vi "Create Interlocked Q Class.vi"(10 "Process State Data":refnum<data-value>, 11 "Process Q":refnum<class "Message Enqueuer.lvclass">) -> (3 "Interlock Q Class out":refnum<class "Interlock Q Class.lvclass">)   [LabVIEW 2022 SP3, in "Interlock Q Class.lvclass"]
uses:
  Interlock Q Class.lvclass
  <vilib>/ActorFramework/Message Enqueuer/Message Enqueuer.lvclass
  Process State Data/Process State Data.lvclass
  Interlock Q Class.lvclass/Interlock Q Class.ctl
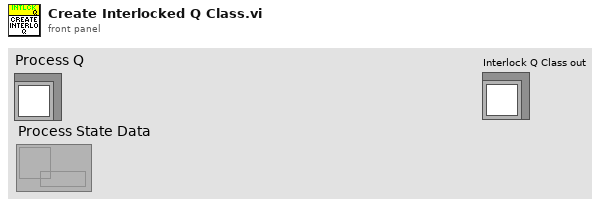
[diagram p1: front panel]
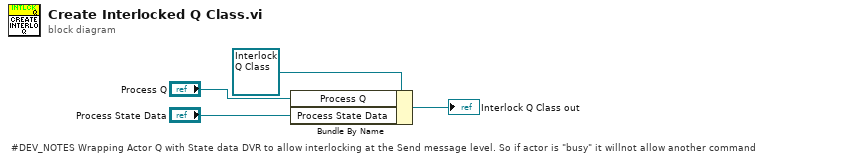
[diagram p0: block diagram]
diagram:
  # "#DEV_NOTES Wrapping Actor Q with State data DVR to allow interlocking at the Send message level. So if actor is \"busy\" it willnot allow another command"
  n1 = Bundle By Name(cluster=refnum<class "Interlock Q Class.lvclass"> refnum ("Interlock Q Class in"), "Process Q"="Process Q", "Process State Data"="Process State Data") -> (→"Interlock Q Class out":refnum<class "Interlock Q Class.lvclass">)
